vi "UpdateAngles.vi"(8 "error in (no error)":errorcluster, 9 "Values":dbl[](array[numeric]), 10 "Angles":dbl[](array[numeric]), 11 "LinearInterpolation in":refnum<class "LinearInterpolation.lvclass">) -> (0 "error out":errorcluster, 3 "LinearInterpolation out":refnum<class "LinearInterpolation.lvclass">)   [LabVIEW 2012, in "LinearInterpolation.lvclass"]
doc: "Takes in new angle-value pairs and inputs them for use in future angle calculations from the linear interpreter."
uses:
  LinearInterpolation.lvclass
  LinearInterpolation.lvclass/LinearInterpolation.ctl
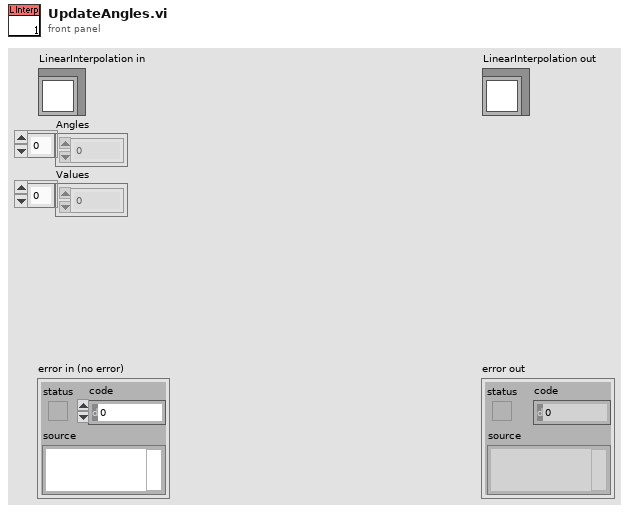
[diagram p1: front panel]
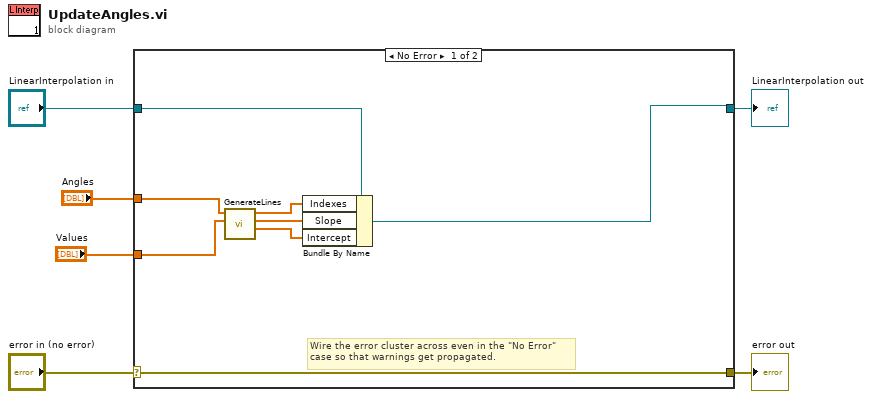
[diagram p0: block diagram]
diagram:
  n1 = case shown="No Error" "error in (no error)" {
    selector: "error in (no error)" -> [w14 w16]
    tunnel: [w14 w16] -> w5
    tunnel: [w12 w15] -> w3
    tunnel: "LinearInterpolation in" -> [w13 w15]
    tunnel: "Values" -> [w10 _]
    tunnel: "Angles" -> [w11 _]
    frame No Error {
      # "Wire the error cluster across even in the \"No Error\"\ncase so that warnings get propagated."
      n2 = call "GenerateLines.vi"("Values"=w10, "Angles"=w11) -> ("Intercept"=w7:dbl[], "Slope"=w8:dbl[], "Angles/Indicies"=w9:dbl[])  [unwired: 7 in]
      n3 = Bundle By Name(cluster=w13, "Indexes"=w9, "Slope"=w8, "Intercept"=w7) -> (w12:refnum<class "LinearInterpolation.lvclass">)
    }
    frame Error {
    }
  }
  "error out" <- w5
  "LinearInterpolation out" <- w3
